vi "Get Application Refs.vi"(8 "Error In":errorcluster, 11 "Application in":refnum<vi>) -> (0 "Error Out":errorcluster, 2 "Owning Project":refnum<vi>, 3 "Application out":refnum<vi>)   [LabVIEW 2019, in "VI Scripting Tools.lvlib"]
uses:
  VI Scripting Tools.lvlib
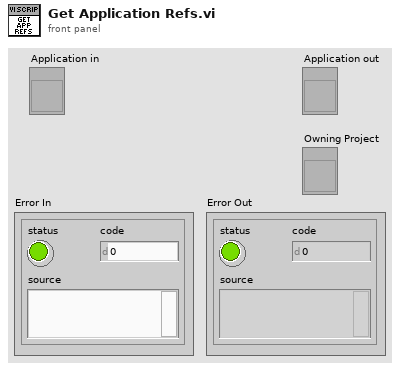
[diagram p1: front panel]
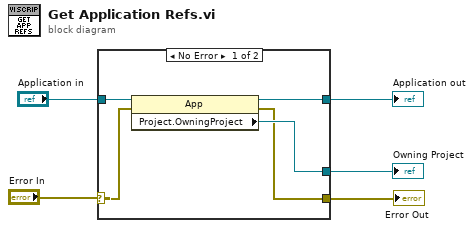
[diagram p0: block diagram]
diagram:
  n1 = case shown="No Error" "Error In" {
    selector: "Error In" -> [w7 w11]
    tunnel: [w10 _] -> w5
    tunnel: [w9 w12] -> w4
    tunnel: "Application in" -> [w8 w12]
    tunnel: [w6 w11] -> w1
    frame No Error {
      n2 = property class="App"(reference=w8, error in=w7) -> (reference out=w9:refnum<vi>, error out=w6:errorcluster, "Project.OwningProject"=w10:refnum<vi>)
    }
    frame Error {
    }
  }
  "Owning Project" <- w5
  "Application out" <- w4
  "Error Out" <- w1
